vi "Destroy.vi"(0 "reference in":refnum<class "BrowerComponent.lvclass">, 5 "error in (no error)":errorcluster) -> (14 "reference out":refnum<class "BrowerComponent.lvclass">, 19 "error out":errorcluster)   [LabVIEW 2015, in "BrowerComponent.lvclass"]
uses:
  BrowerComponent.lvclass
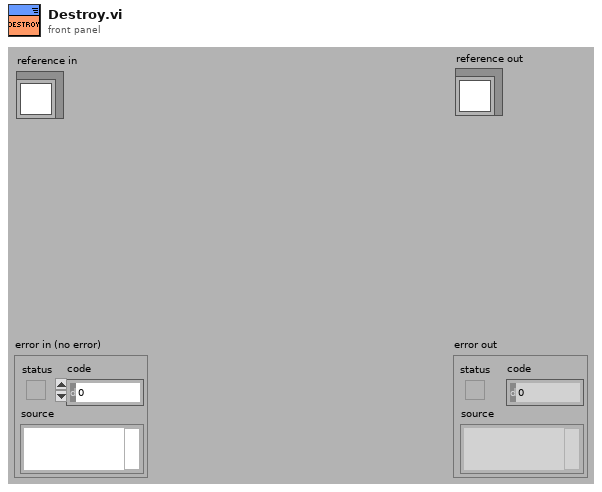
[diagram p1: front panel]
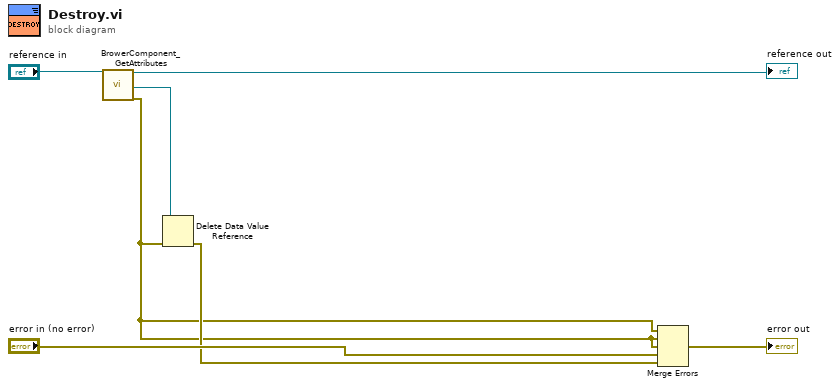
[diagram p0: block diagram]
diagram:
  n1 = call "BrowerComponent_GetAttributes.vi"("reference in"="reference in") -> ("reference out"=→"reference out":refnum<class "BrowerComponent.lvclass">, "DataRef"=w4:refnum<data-value>, "error out"=w1:errorcluster)  [unwired: 15 in, 1 out]
  n2 = Delete Data Value Reference(data value reference=w4, error in=w1) -> (error out=w2:errorcluster)  [unwired: 1 out]
  n3 = Merge Errors(w1, w1, w1, "error in (no error)", w2) -> (→"error out":errorcluster)
